vi "挖开周围地块.vi"(0 "地图":i32[][](array[numeric]), 1 "索引":i32) -> (2 "输出地图":i32[][](array[numeric]), 3 "对话框信息":string, 4 "胜利失败":bool, 5 "游戏结束":bool)   [LabVIEW 2017]
panel:
  out "数组":i32[](array[numeric])
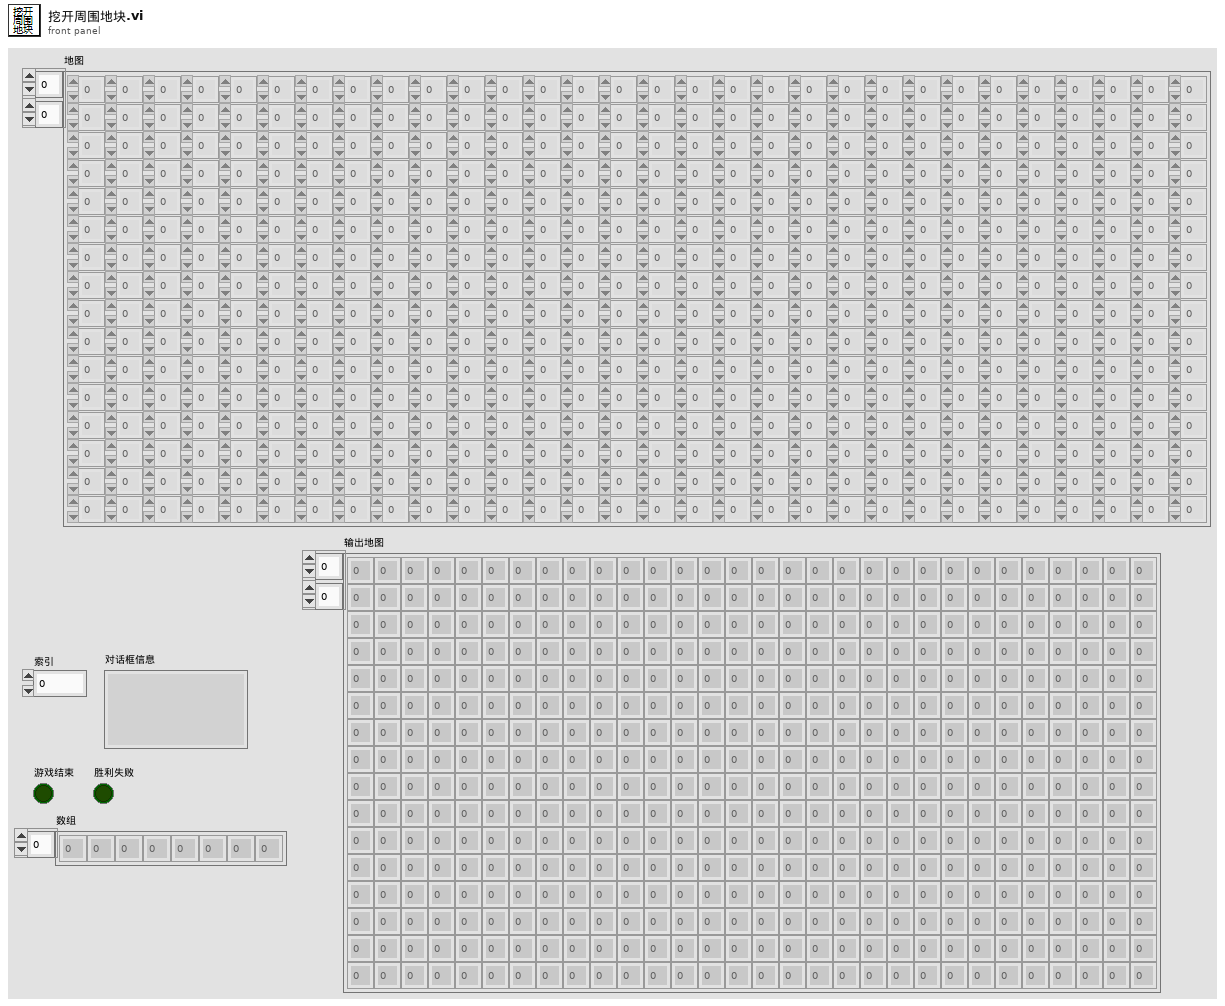
[diagram p1: front panel]
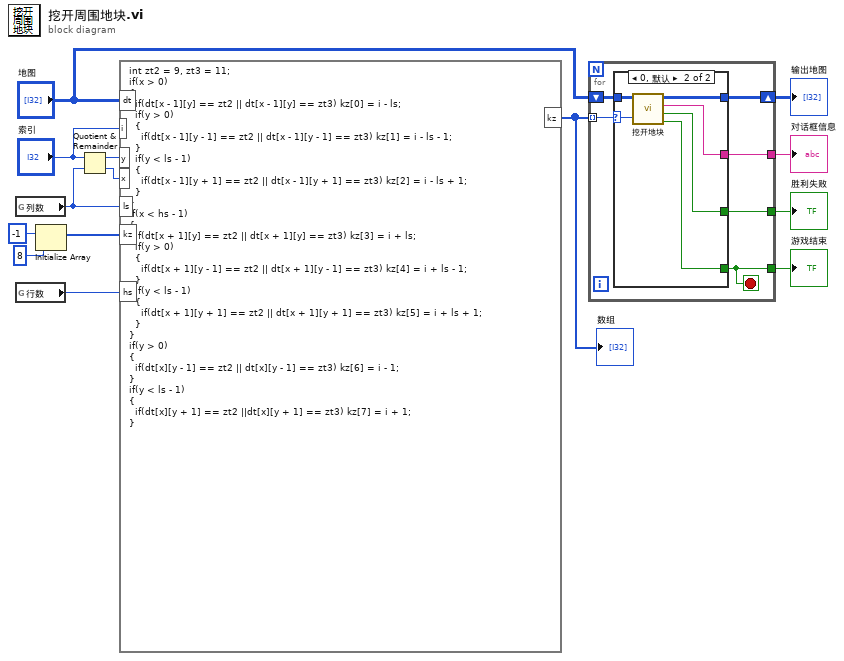
[diagram p0: block diagram]
diagram:
  n1 = global read "全局变量.vi" "列数"() -> (w2:i32)
  n2 = global read "全局变量.vi" "行数"() -> (w1:i32)
  n3 = Initialize Array(-1, 8 ("维数大小")) -> (w10:i32[])
  n4 = Quotient & Remainder(x="索引", y=w2) -> (x-y*floor(x/y)=w13:i32, floor(x/y)=w14:i32)
  n5 = formula code="int zt2 = 9, zt3 = 11;\nif(x > 0)\n{\n  if(dt[x - 1][y] == zt2 || dt[x - 1][y] == zt3) kz[0] = i - ls;\n  if(y > 0)\n  {\n    if(dt[x - 1][y - 1] == zt2 || dt[x - 1][y - 1] == zt3) kz[1] = i - ls - 1;\n  }\n  if(y < ls - 1)\n  {\n    if(dt[x - 1][y + 1] == zt2 || dt[x - 1][y + 1] == zt3) kz[2] = i - ls + 1;\n  }\n}\nif(x < hs - 1)\n{\n  if(dt[x + 1][y] == zt2 || dt[x + 1][y] == zt3) kz[3] = i + ls;\n  if(y > 0)\n  {\n    if(dt[x + 1][y - 1] == zt2 || dt[x + 1][y - 1] == zt3) kz[4] = i + ls - 1;\n  }\n  if(y < ls - 1)\n  {\n    if(dt[x + 1][y + 1] == zt2 || dt[x + 1][y + 1] == zt3) kz[5] = i + ls + 1;\n  }\n}\nif(y > 0)\n{\n  if(dt[x][y - 1] == zt2 || dt[x][y - 1] == zt3) kz[6] = i - 1;\n}\nif(y < ls - 1)\n{\n  if(dt[x][y + 1] == zt2 ||dt[x][y + 1] == zt3) kz[7] = i + 1;\n}"("dt"="地图", "y"=w13, "x"=w14, "kz"=w10, "i"="索引", "ls"=w2, "hs"=w1) -> ("kz"=w5:i32[])
  "数组" <- w5
  n6 = for {
    tunnel: w5 -> [w20] mode=indexing
    tunnel: [w19] -> w8
    tunnel: [w18] -> w7
    tunnel: [w17] -> w6
    shift-right: [w16] -> w4
    shift-left: "地图" -> [w15]
    stop <- w17 stop-if-true
    n7 = case shown="0, 默认" w20 {
      selector: w20 -> [_ w27]
      tunnel: [_ w26] -> w17
      tunnel: [_ w25] -> w19
      tunnel: [_ w24] -> w18
      tunnel: [w21 w22] -> w16
      tunnel: w15 -> [w21 w23]
      frame -1 {
      }
      frame 0, Default {
        n8 = call "挖开地块.vi"("地图"=w23, "索引"=w27) -> ("输出地图"=w22:i32[][], "对话框信息"=w25:string, "胜利失败"=w24:bool, "游戏结束"=w26:bool)
      }
    }
  }
  "游戏结束" <- w6
  "胜利失败" <- w7
  "输出地图" <- w4
  "对话框信息" <- w8
